vi "菜单-编译.vi"(8 "error in (no error)":errorcluster caption="错误输入（无错误）", 11 "程序响应 输入":refnum<class "程序响应.lvclass">) -> (0 "error out":errorcluster caption="错误输出", 3 "程序响应 输出":refnum<class "程序响应.lvclass">)   [LabVIEW 2018, in "程序响应.lvlib" / "程序响应.lvclass"]
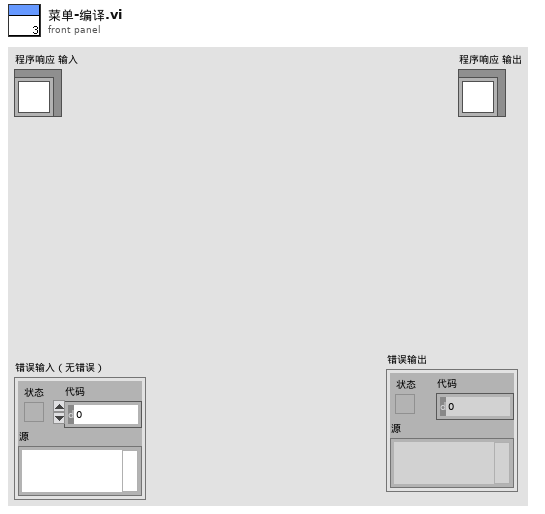
[diagram p1: front panel]
types:
  T1 = enum16{"open", "replace", "create", "open or create", "replace or create", "replace or create with confirmation"}
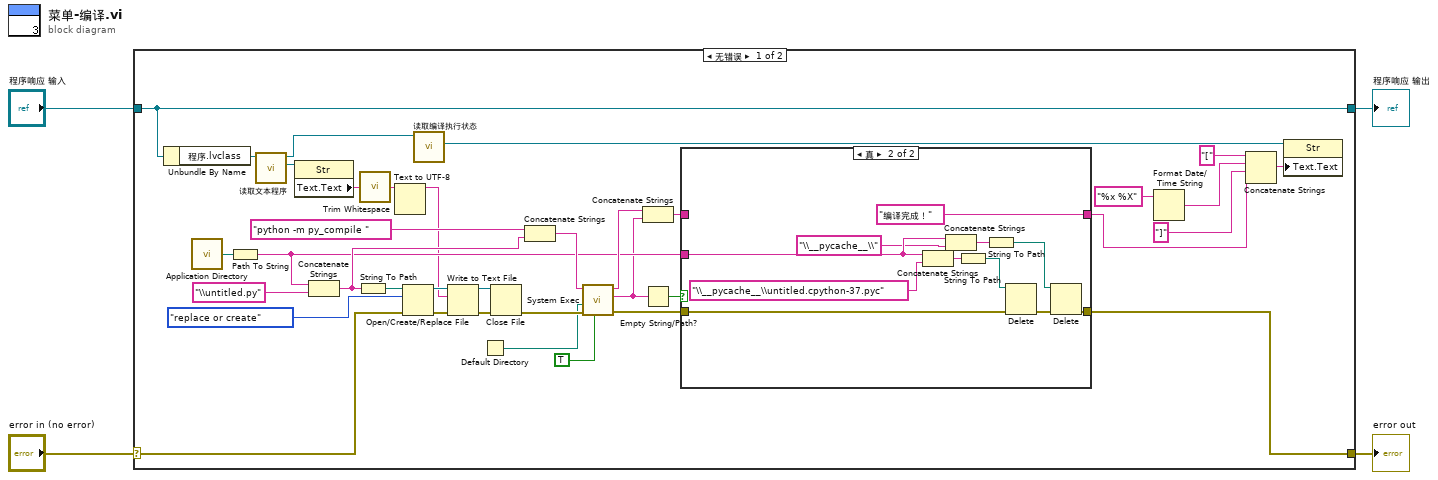
[diagram p0: block diagram]
diagram:
  n1 = case shown="无错误" "error in (no error)" {
    selector: "error in (no error)" -> [w18 w55]
    tunnel: [w17 w55] -> w3
    tunnel: [w23 w54] -> w1
    tunnel: "程序响应 输入" -> [w23 w54]
    frame No Error {
      n2 = Unbundle By Name(w23) -> ("程序.lvclass"=w40:refnum<class "程序.lvclass">)
      n3 = call <vilib>:"Application Directory.vi"() -> ("Application Directory"=w37:path)
      n4 = Path To String(path=w37) -> (string=w16:string)
      n5 = call-dynamic "读取文本程序.vi"("程序输入"=w40) -> ("文本程序"=w39:refnum<vi>, "程序输出"=w20:refnum<class "程序.lvclass">)  [unwired: 8 in, 1 out]
      n6 = property class="Str"(reference=w39) -> ("Text.Text"=w38:string)  [unwired: 1 in, 2 out]
      n7 = Concatenate Strings(w16, "\\untitled.py" ("字符串")) -> (w28:string)
      n8 = String To Path(string=w28) -> (path=w35:path)
      n9 = call <vilib>:"Trim Whitespace.vi"("string"=w38) -> ("trimmed string"=w6:string)  [unwired: 1 in]
      n10 = Text to UTF-8 ("文本至UTF-8转换")(11:w6) -> (3:w5:string)  [unwired: 2 in, 1 out]
      n11 = Open/Create/Replace File(file path (use dialog)=w35, error in=w18, operation (0:open)=T1."replace or create" ("操作(0:open)")) -> (refnum out=w34:refnum<file>, error out=w33:errorcluster)  [unwired: 3 in, 1 out]
      n12 = call-dynamic "读取编译执行状态.vi"("程序输入"=w20) -> ("编译执行状态"=w19:refnum<vi>)  [unwired: 8 in, 2 out]
      n13 = Write to Text File(file (use dialog)=w34, text=w5, error in=w33) -> (refnum out=w32:refnum<file>, error out=w31:errorcluster)  [unwired: 1 in, 1 out]
      n14 = Default Directory() -> (w24:path)
      n15 = Close File(refnum=w32, error in=w31) -> (error out=w29:errorcluster)  [unwired: 1 out]
      n16 = Concatenate Strings("python -m py_compile " ("字符串"), w28) -> (w27:string)
      n17 = call <vilib>:"System Exec.vi"("run minimized? (F)"=TRUE, "error in (no error)"=w29, "working directory"=w24, "command line"=w27) -> ("error out"=w26:errorcluster, "standard error"=w15:string, "standard output"=w25:string)  [unwired: 4 in, 1 out]
      n18 = Concatenate Strings(w25, w15) -> (w13:string)
      n19 = Empty String/Path?(string/path=w15) -> (empty?=w14:bool)
      n20 = case shown="真" w14 {
        tunnel: w26 -> [w42 w53]
        tunnel: [w42 w48] -> w17
        tunnel: w16 -> [_ w47]
        tunnel: w13 -> [w41 _]
        tunnel: [w41 "编译完成！"] -> w8
        frame False {
          # "编译不通过"
        }
        frame True {
          n21 = Concatenate Strings(w47, "\\__pycache__\\untitled.cpython-37.pyc" ("字符串")) -> (w51:string)
          n22 = Concatenate Strings(w47, "\\__pycache__\\" ("字符串")) -> (w45:string)
          n23 = String To Path(string=w51) -> (path=w50:path)
          n24 = String To Path(string=w45) -> (path=w44:path)
          n25 = Delete(path (use dialog)=w50, error in=w53) -> (error out=w49:errorcluster)  [unwired: 3 in, 2 out]
          n26 = Delete(path (use dialog)=w44, error in=w49) -> (error out=w48:errorcluster)  [unwired: 3 in, 2 out]
        }
      }
      n27 = Format Date/Time String(time format string (%c)="%x %X" ("时间格式字符串(%c)")) -> (date/time string=w9:string)  [unwired: 2 in]
      n28 = Concatenate Strings("[" ("字符串"), w9, "]" ("字符串"), w8) -> (w7:string)
      n29 = property class="Str"(reference=w19, "Text.Text"=w7) -> ()  [unwired: 1 in, 2 out]
    }
    frame Error {
    }
  }
  "error out" <- w3
  "程序响应 输出" <- w1
